vi "MoveFile.vi"(8 "error in":errorcluster, 11 "File Name":string) -> (0 "error out":errorcluster)   [LabVIEW 2019]
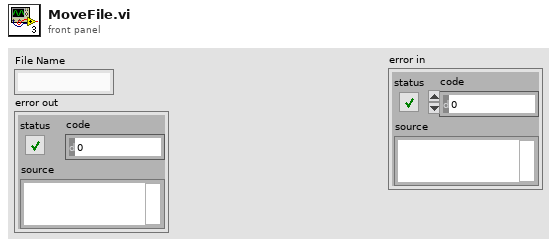
[diagram p1: front panel]
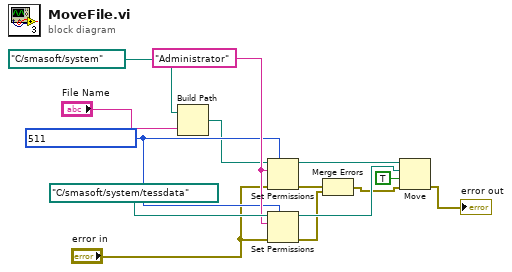
[diagram p0: block diagram]
diagram:
  w9 = i16 511 ("permissions")
  w10 = "Administrator" ("new owner")
  n1 = Build Path(base path=path "C:/smasoft/system" ("source path"), name or relative path="File Name") -> (appended path=w6:path)
  n2 = Set Permissions(7:w9, 8:"error in", 10:w10, 11:w6) -> (0:w5:errorcluster, 3:w13:path)  [unwired: 1 in]
  n3 = Set Permissions(7:w9, 8:"error in", 10:w10, 11:path "C:/smasoft/system/tessdata" ("source path 2")) -> (0:w4:errorcluster, 3:w11:path)  [unwired: 1 in]
  n4 = Merge Errors(w5, w4) -> (w3:errorcluster)
  n5 = Move(source path=w13, error in=w3, 9:TRUE ("overwrite (F)"), 10:w11) -> (error out=→"error out":errorcluster)  [unwired: 1 in, 2 out]
